vi "pp2_DAQwritePlayClick.vi"(0 "State In":T1={"Curr  tr"=0, "Curr (ms)"=0, "Cum (ms)"=0, "Run loop diff"=0, "Tone countdown (ms)"=0, "Countdown (ms)"=0, "Curr State"=enum."0 NULL", "Prev State"=enum."1 Habituation", "Rw"=FALSE, "Sw"=FALSE, "Tone\nGate"=FALSE, "Punish"=FALSE, "Current DAQ DO Int"=0, "Current Loaded Trial"={"Trial Type Number"=1, "Trial Type"=enum."GO", "Trial Weight"=100, "Shock (mA)"=0.3, "Duration (ms)"=0.25, "Sound Type"=enum."04 FM Sweep", "Stim P1"=4000.0, "Stim P2"=0.0, "Stim P3"=0.0, "Stim P4"=2000.0}, "Next Trial (for display purposes)"={"Trial Type Number"=1, "Trial Type"=enum."GO", "Trial Weight"=100, "Shock (mA)"=0.3, "Duration (ms)"=0.25, "Sound Type"=enum."04 FM Sweep", "Stim P1"=4000.0, "Stim P2"=0.0, "Stim P3"=0.0, "Stim P4"=2000.0}, "Total trials memo"=0, "State start cum memo (ms)"=0, "Last dur jump time memo (ms)"=0, "Last dur shock time memo (ms)"=0, "Tone repeat memo (ms)"=0, "Webcam on"=FALSE, "Webcam recording"=FALSE, "State update flag"=FALSE, "Last loaded shock voltage"=0.0, "Vid upd"=enum."0"} {"Current DAQ DO Int" format="%016b"; "Next Trial (for display purposes)"."Shock (mA)" min=-1.0 max=5.0; "Next Trial (for display purposes)"."Trial Weight" step=1; "Next Trial (for display purposes)"."Duration (ms)" min=0.0 max=1.0; "Next Trial (for display purposes)"."Trial Type Number" min=1 max=256 step=1; "Current Loaded Trial"."Shock (mA)" min=-1.0 max=5.0; "Current Loaded Trial"."Trial Weight" step=1; "Current Loaded Trial"."Duration (ms)" min=0.0 max=1.0; "Current Loaded Trial"."Trial Type Number" min=1 max=256 step=1}, 1 "Daq config":T6={"Sound AO"="Dev2/ao0", "Shock intesity AO"="Dev1/ao1", "Code_LED DO"="Dev1/port1:2", "Switch DI"="Dev1/port0/line0:1", "Webcam"="cam0", "Sound AO task"="", "Sound card task"=0, "Shock intensity AO task"="", "Code_LED DO task"="", "Switch DI task"="", "AO <=> Sound card"=FALSE, "Sound card"=0, "sample rate"=8000.0, "Variable shock"=FALSE, "Webcam on"=FALSE, "Tone gate PFI"="/Dev1/PFI1", "Waveform memo"={"t0"=timestamp(0 s since 1904-01-01), "dt"=1.0, "Y"=[]}, "First time"=FALSE} {"sample rate" min=8000.0; "Sound card task" format="%.0x"}, 2 "Pre click \n(V)":dbl, 3 "error in (no error)":errorcluster) -> (8 "Daq config 2":T6={"Sound AO"="Dev2/ao0", "Shock intesity AO"="Dev1/ao1", "Code_LED DO"="Dev1/port1:2", "Switch DI"="Dev1/port0/line0:1", "Webcam"="cam0", "Sound AO task"="", "Sound card task"=0, "Shock intensity AO task"="", "Code_LED DO task"="", "Switch DI task"="", "AO <=> Sound card"=FALSE, "Sound card"=0, "sample rate"=8000.0, "Variable shock"=FALSE, "Webcam on"=FALSE, "Tone gate PFI"="/Dev1/PFI1", "Waveform memo"={"t0"=timestamp(0 s since 1904-01-01), "dt"=1.0, "Y"=[]}, "First time"=FALSE} {"sample rate" min=8000.0; "Sound card task" format="%.0x"}, 10 "error out":errorcluster)   [LabVIEW 2013]
uses:
  pp2_CTL_DaqConfig.ctl
  <vilib>/userdefined/High Color/IMAQdx.ctl
  <vilib>/sound2/lvsound2.llb/Sound Output Task ID.ctl
  pp2_CTL_StateInfo.ctl
  pp2_CTL_State.ctl
  pp2_CTL_Trial.ctl
  pp2_CTL_TrialType.ctl
  labolabo2/waveforms/WFTypes.ctl
  <vilib>/sound2/lvsound2.llb/Sound Output Write (DBL Single).vi
  <vilib>/DAQmx/create/channels.llb/DAQmx Create Channel (AO-Voltage-Basic).vi
  <vilib>/DAQmx/configure/timing.llb/DAQmx Timing (Use Waveform).vi
  <vilib>/DAQmx/write.llb/DAQmx Write (Analog Wfm 1Chan NSamp).vi
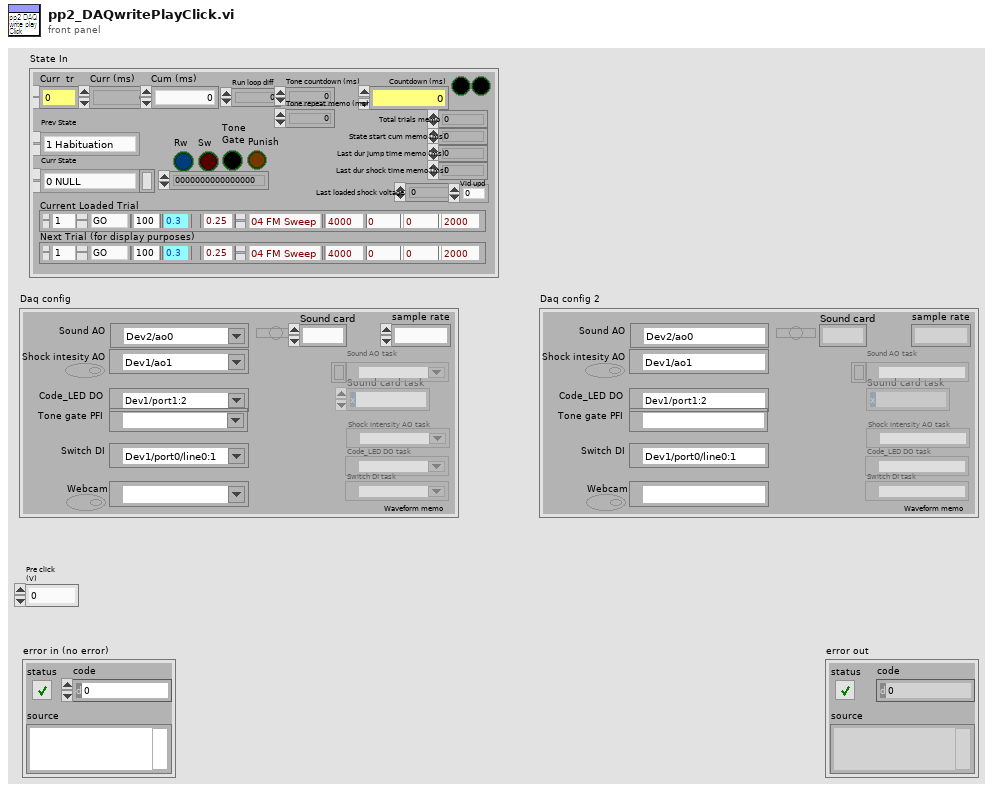
[diagram p1: front panel]
types:
  T1 = typedef "pp2_CTL_StateInfo.ctl" = cluster{"Curr  tr":u16, "Curr (ms)":u32, "Cum (ms)":i64, "Run loop diff":i64, "Tone countdown (ms)":i64, "Countdown (ms)":i64, "Curr State":T2, "Prev State":T2, "Rw":bool, "Sw":bool, "Tone\nGate":bool, "Punish":bool, "Current DAQ DO Int":u16, "Current Loaded Trial":T3, "Next Trial (for display purposes)":T3, "Total trials memo":i64, "State start cum memo (ms)":i64, "Last dur jump time memo (ms)":i64, "Last dur shock time memo (ms)":i64, "Tone repeat memo (ms)":i64, "Webcam on":bool, "Webcam recording":bool, "State update flag":bool, "Last loaded shock voltage":dbl, "Vid upd":enum16{"0", "1", "2", "3", "4", "5", "6", "7", "8", "9"}}
  T2 = typedef "pp2_CTL_State.ctl" = enum8{"0 NULL", "1 Habituation", "2 (Load Trial)", "3 Stay Period", "4 Load Audio/Click Delay", "5 GO Trial", "6 GO Jumped", "7 GO Timeout", "8 NOGO Trial", "9 NOGO Jumped", "10 NOGO Timeout", "11 TEST Trial", "12 TEST Jumped", "13 TEST Timeout", "14 Intertrial Interval", "15 Done"}
  T3 = typedef "pp2_CTL_Trial.ctl" = cluster{"Trial Type Number":i16, "Trial Type":T4, "Trial Weight":u32, "Shock (mA)":dbl, "Duration (ms)":dbl, "Sound Type":T5, "Stim P1":dbl, "Stim P2":dbl, "Stim P3":dbl, "Stim P4":dbl}
  T4 = typedef "pp2_CTL_TrialType.ctl" = enum16{"OFF", "GO", "NOGO", "TEST"}
  T5 = typedef "WFTypes.ctl" = enum16{"00 NULL", "01 DC", "02 Noise", "03 Pure Tone", "04 FM Sweep"}
  T6 = typedef "pp2_CTL_DaqConfig.ctl" = cluster{"Sound AO":tag, "Shock intesity AO":tag, "Code_LED DO":tag, "Switch DI":tag, "Webcam":T7, "Sound AO task":refnum<k21>, "Sound card task":T8, "Shock intensity AO task":refnum<k21>, "Code_LED DO task":refnum<k21>, "Switch DI task":refnum<k21>, "AO <=> Sound card":bool, "Sound card":u32, "sample rate":dbl, "Variable shock":bool, "Webcam on":bool, "Tone gate PFI":tag, "Waveform memo":waveform(dbl), "First time":bool}
  T7 = typedef "IMAQdx.ctl" = refnum<k21>
  T8 = typedef "Sound Output Task ID.ctl" = u32
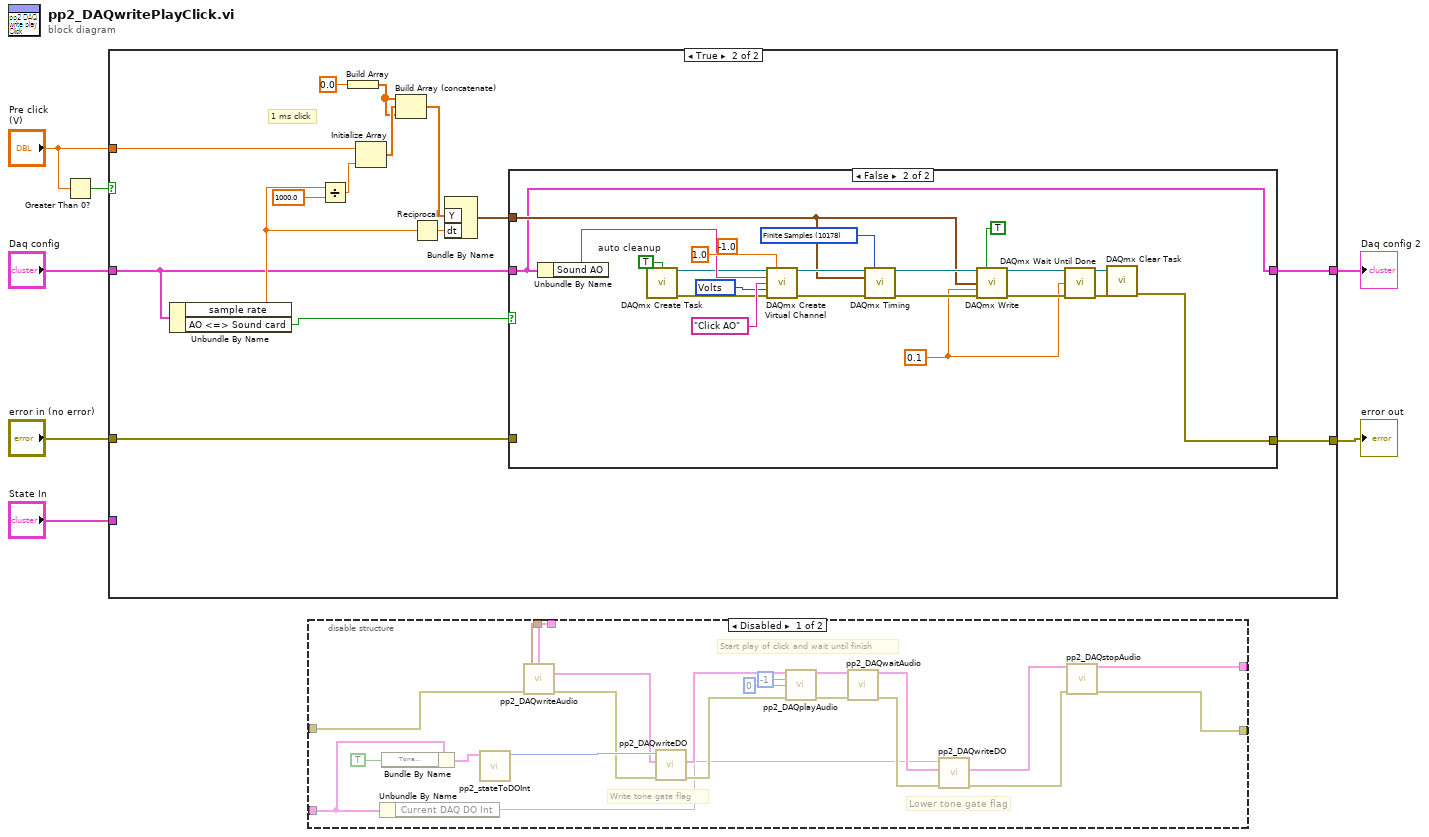
[diagram p0: block diagram]
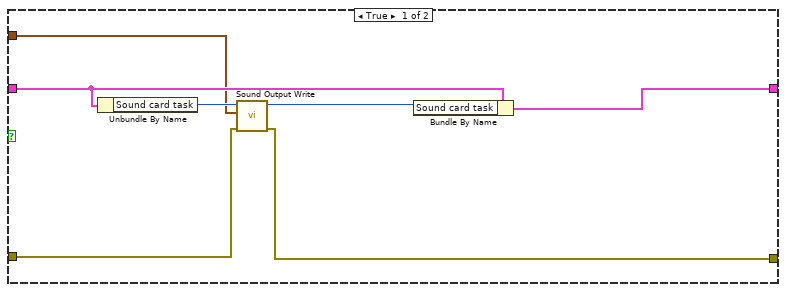
[diagram p4: hidden frame]
diagram:
  n1 = Greater Than 0?(x="Pre click \n(V)") -> (x > 0?=w3:bool)
  n2 = case shown="True" w3 {
    tunnel: "error in (no error)" -> [w8 w24]
    tunnel: [w8 w22] -> w6
    tunnel: [w9 w23] -> w5
    tunnel: "Daq config" -> [w9 w11]
    tunnel: "Pre click \n(V)" -> [_ w13]
    tunnel: "State In" -> [_ _]
    frame False {
      # "If click amplitude is negative or zero, then just pass through without anything"
    }
    frame True {
      # "1 ms click"
      n3 = Unbundle By Name(w11) -> ("sample rate"=w16:dbl, "AO <=> Sound card"=w12:bool)
      n4 = Divide(x=w16, y=1000.0) -> (x/y=w18:dbl)
      n5 = Build Array(0.0 ("element")) -> (w19:dbl[])
      n6 = Initialize Array(w13, w18) -> (w21:dbl[])
      n7 = Build Array (concatenate)(w19, w21, w19) -> (w20:dbl[])
      n8 = Reciprocal(x=w16) -> (1/x=w15:dbl)
      n9 = Bundle By Name("Y"=w20, "dt"=w15) -> (w10:waveform(dbl))  [unwired: 1 in]
      n10 = case shown="False" w12 {
        tunnel: w24 -> [w30 _]
        tunnel: [w31 w32] -> w23
        tunnel: [w29 w35] -> w22
        tunnel: w11 -> [w26 w32]
        tunnel: w10 -> [w25 w34]
        frame True {
          n11 = Unbundle By Name(w26) -> ("Sound card task"=w27:T8)
          n12 = call-poly <vilib>:"Sound Output Write.vi"("error in (no error)"=w30, "data"=w25, "task ID"=w27) -> ("error out"=w29:errorcluster, "task ID out"=w28:T8)  [unwired: 7 in]
          n13 = Bundle By Name(cluster=w26, "Sound card task"=w28) -> (w31:T6)
        }
        frame False {
          w33 = 0.1 ("timeout")
          w38 = TRUE  # auto cleanup
          w48 = 10178 items=["Finite Samples"=10178, "Continuous Samples"=10123, "Hardware Timed Single Point"=12522] ("sample mode")
          w50 = 10348 items=["Volts"=10348, "From Custom Scale"=10065] ("units")
          (unwired) -1.0 ("minimum value")
          n14 = Unbundle By Name(w32) -> ("Sound AO"=w49:tag)
          n15 = call <vilib>:"DAQmx Create Task.vi"("auto cleanup"=w38) -> ("task out"=w37:refnum<k21>, "error out"=w36:errorcluster)  [unwired: 13 in]
          n16 = call-poly <vilib>:"DAQmx Create Virtual Channel.vi"("task in"=w37, "maximum value"=1.0, "physical channels"=w49, "name to assign"="Click AO", "units"=w50, "error in"=w36) -> ("task out"=w47:refnum<k21>, "error out"=w46:errorcluster)  [unwired: 8 in]
          n17 = call-poly <vilib>:"DAQmx Timing.vi"("task/channels in"=w47, "sample mode"=w48, "waveform"=w34, "error in"=w46) -> ("task out"=w45:refnum<k21>, "error out"=w44:errorcluster)  [unwired: 10 in]
          n18 = call-poly <vilib>:"DAQmx Write.vi"("task/channels in"=w45, "auto start"=TRUE, "data"=w34, "timeout"=w33, "error in"=w44) -> ("task out"=w42:refnum<k21>, "error out"=w41:errorcluster)  [unwired: 8 in, 1 out]
          n19 = call <vilib>:"DAQmx Wait Until Done.vi"("task/channels in"=w42, "timeout (sec)"=w33, "error in"=w41) -> ("task out"=w40:refnum<k21>, "error out"=w39:errorcluster)  [unwired: 11 in]
          n20 = call <vilib>:"DAQmx Clear Task.vi"("task in"=w40, "error in"=w39) -> ("error out"=w35:errorcluster)  [unwired: 13 in]
        }
      }
    }
  }
  "error out" <- w6
  "Daq config 2" <- w5
  n21 = disable-structure shown="Disabled" {
    disable-tunnel: _ -> [w74 _]
    disable-tunnel: _ -> [w73 _]
    disable-tunnel: _ -> [w72 _]
    disable-tunnel: _ -> [w71 _]
    disable-tunnel: [w55 _] -> _
    disable-tunnel: [w53 _] -> _
    frame Disabled {
      # "Start play of click and wait until finish"
      # "Lower tone gate flag"
      # "Write tone gate flag"
      n22 = Unbundle By Name(w74) -> ("Current DAQ DO Int"=w59)
      n23 = Bundle By Name(cluster=w74, "Tone\nGate"=TRUE ("Tone\nGate")) -> (w70:cluster{})
      n24 = call "pp2_stateToDOInt.vi"("State In"=w70) -> ("DAQ Output Int"=w68:u16)  [unwired: 10 in]
      n25 = call "pp2_DAQwriteAudio.vi"("Daq config In"=w71, "Waveform"=w73, "error in (no error)"=w72) -> ("Daq config Out"=w58:T6, "error out"=w57:errorcluster)  [unwired: 11 in]
      n26 = call "pp2_DAQwriteDO.vi"("error in (no error)"=w57, "Daq config"=w58, "DAQ Digital In"=w68) -> ("error out"=w66:errorcluster, "Daq config 2"=w67:T6)  [unwired: 7 in]
      n27 = call "pp2_DAQplayAudio.vi"("Daq config In"=w67, "State In"=i64 -1 ("Tone countdown (ms) In"), 7:i64 0 ("Tone repeat memo"), "error in (no error)"=w66) -> ("Daq config Out"=w63:T6, "error out"=w62:errorcluster)  [unwired: 9 in, 1 out]
      n28 = call "pp2_DAQwaitAudio.vi"("Daq config In"=w63, "error in (no error)"=w62) -> ("Daq config Out"=w60:T6, "error out"=w61:errorcluster)  [unwired: 12 in]
      n29 = call "pp2_DAQwriteDO.vi"("error in (no error)"=w61, "Daq config"=w60, "DAQ Digital In"=w59) -> ("error out"=w54:errorcluster, "Daq config 2"=w56:T6)  [unwired: 7 in]
      n30 = call "pp2_DAQstopAudio.vi"("Daq config In"=w56, "error in (no error)"=w54) -> ("Daq config Out"=w55:T6, "error out"=w53:errorcluster)  [unwired: 12 in]
    }
    frame Enabled {
    }
  }
